vi "Time Tag to Time Stamp.vi"(9 "day of year":u32, 10 "buffer report word":u32, 11 "time tag":u32 format="%x") -> (2 "ns counter":u64, 3 "time stamp":timestamp)   [LabVIEW 2020, in "AIM ARINC 429 Hardware API.lvlib"]
doc: "Time tag to time stamp."
uses:
  <vilib>/Utility/miscctls.llb/LVDateTimeRec.ctl
  AIM ARINC 429 Hardware API.lvlib
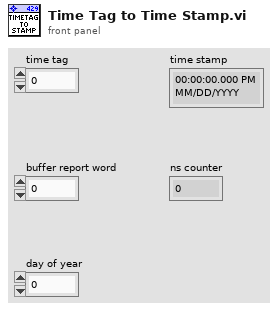
[diagram p1: front panel]
types:
  T1 = typedef "LVDateTimeRec.ctl" = cluster{"fractional second":dbl, "second":i32, "minute":i32, "hour":i32, "day of month":i32, "month":i32, "year":i32, "day of week":i32, "day of year":i32, "DST":i32}
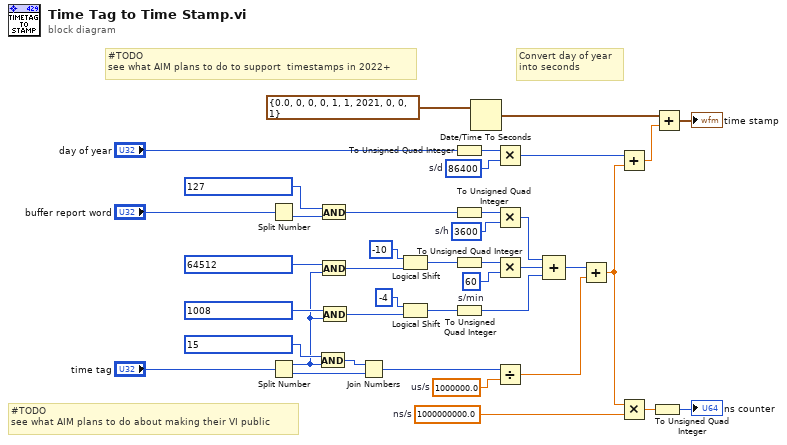
[diagram p0: block diagram]
diagram:
  w9 = u64 3600  # s/h
  w16 = u64 86400  # s/d
  w25 = 1000000000.0  # ns/s
  w30 = u64 60  # s/min
  w40 = 1000000.0  # us/s
  # "#TODO\nsee what AIM plans to do to support  timestamps in 2022+"
  # "#TODO\nsee what AIM plans to do about making their VI public"
  # "Convert day of year into seconds"
  n1 = Split Number(x="buffer report word") -> (lo(x)=w21:u16)  [unwired: 1 out]
  n2 = Split Number(x="time tag") -> (hi(x)=w23:u16, lo(x)=w24:u16)
  n3 = And(x=u16 15, y=w23) -> (x .and. y?=w38:u16)
  n4 = And(x=u16 127, y=w21) -> (x .and. y?=w14:u16)
  n5 = And(x=u16 64512, y=w23) -> (x .and. y?=w33:u16)
  n6 = And(x=u16 1008, y=w23) -> (x .and. y?=w35:u16)
  n7 = Join Numbers(hi=w38, lo=w24) -> ((hi.lo)=w27:u32)
  n8 = Logical Shift(y=i16 -10, x=w33) -> (x << y=w31:u16)
  n9 = Logical Shift(y=i16 -4, x=w35) -> (x << y=w28:u16)
  n10 = To Unsigned Quad Integer(1:"day of year") -> (0:w10:u64)
  n11 = To Unsigned Quad Integer(1:w14) -> (0:w8:u64)
  n12 = To Unsigned Quad Integer(1:w31) -> (0:w7:u64)
  n13 = To Unsigned Quad Integer(1:w28) -> (0:w6:u64)
  n14 = Date/Time To Seconds(2:T1 {"fractional second"=0.0, "second"=0, "minute"=0, "hour"=0, "day of month"=1, "month"=1, "year"=2021, "day of week"=0, "day of year"=0, "DST"=1} ("date time rec")) -> (0:w12:timestamp)  [unwired: 1 in]
  n15 = Multiply(x=w10, y=w16) -> (x*y=w2:u64)
  n16 = Multiply(x=w8, y=w9) -> (x*y=w13:u64)
  n17 = Multiply(x=w7, y=w30) -> (x*y=w29:u64)
  n18 = Divide(x=w27, y=w40) -> (x/y=w5:dbl)
  n19 = Compound Arithmetic op=ADD(w13, w29, w6) -> (w4:u64)
  n20 = Add(x=w4, y=w5) -> (x+y=w3:dbl)
  n21 = Add(x=w2, y=w3) -> (x+y=w1:dbl)
  n22 = Multiply(x=w3, y=w25) -> (x*y=w26:dbl)
  n23 = To Unsigned Quad Integer(1:w26) -> (0:→"ns counter":u64)
  n24 = Add(x=w12, y=w1) -> (x+y=→"time stamp":timestamp)
